vi "Write Cmd.vi"(8 "error in":errorcluster, 10 "CmdStruct":T1, 11 "3022A in":refnum<class "3022A.lvclass">) -> (0 "error out":errorcluster, 2 "Buffer":string, 3 "3022A out":refnum<class "3022A.lvclass">)   [LabVIEW 2014, in "3022A.lvclass"]
uses:
  3022A.lvclass
  CPC.lvclass
  Controls/CmdStruct.ctl
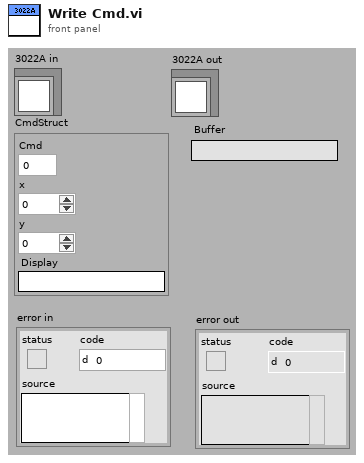
[diagram p1: front panel]
types:
  T1 = typedef "CmdStruct.ctl" = cluster{"Cmd":u8, "x":i64, "y":i64, "Display":string}
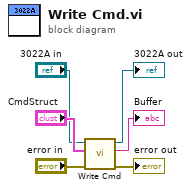
[diagram p0: block diagram]
diagram:
  n1 = call-parent "Write Cmd.vi"("error in"="error in", "CmdStruct"="CmdStruct", "CPC in"="3022A in") -> ("error out"=→"error out":errorcluster, "Buffer"=→"Buffer":string, "CPC out"=→"3022A out":refnum<class "3022A.lvclass">)  [unwired: 6 in]
